vi "Write LIV Test data.vi"(7 "Send any changes now? (F)":bool, 8 "error in (no error)":errorcluster, 10 "LIV Test data":T1(array[cluster]), 11 "Fiber Auto Collimation state data in":refnum<class "Fiber Auto Collimation state data.lvclass">) -> (0 "error out":errorcluster, 3 "Fiber Auto Collimation state data out":refnum<class "Fiber Auto Collimation state data.lvclass">)   [LabVIEW 2018]
doc: "This \"LIV test data\" is just a placeholder and example for how real test data might be stored. This accessor plus its data in the state data class private control probably need to be removed or replaced with something to hold test data for the actual station."
uses:
  Fiber Auto Collimation state data.lvclass
  Tracked state data.ctl
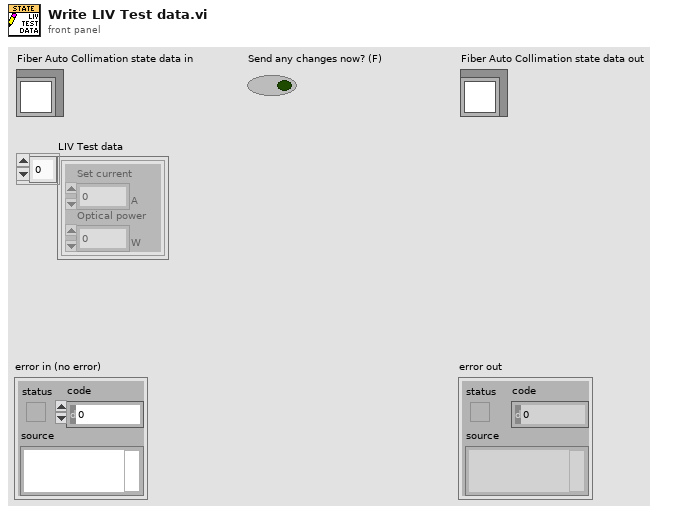
[diagram p1: front panel]
types:
  T1 = cluster{"Set current":sgl[unit], "Optical power":sgl[unit]}[]
  T2 = typedef "Fiber Auto Collimation state data.lvclass/Tracked state data.ctl" = enum16{"No update", "Permission level", "Username", "Test running", "DUT Serial", "Test status", "MOM Lot", "Loaded test recipe", "Model case running", "Station status", "BV data", "Defect Identify data", "Axis Position data", "Fiber Ass PN", "Operator", "RunTime", "VBAI", "Steps Cycle Time"}
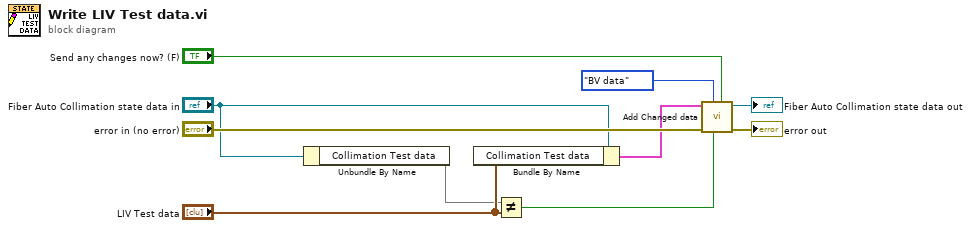
[diagram p0: block diagram]
diagram:
  n1 = Unbundle By Name("Fiber Auto Collimation state data in") -> ("Collimation Test data"=w2)
  n2 = Bundle By Name(cluster="Fiber Auto Collimation state data in", "Collimation Test data"="LIV Test data") -> (w6:cluster{})
  n3 = Not Equal?(x=w2, y="LIV Test data") -> (x != y?=w3:bool)
  n4 = call "Add Changed data.vi"("Send any changes now? (F)"="Send any changes now? (F)", "Data changed?"=w3, "Data type"=Tracked_state_data."BV data", "error in (no error)"="error in (no error)", "Fiber Auto Collimation state data in"=w6) -> ("error out"=→"error out":errorcluster, "Fiber Auto Collimation state data out"=→"Fiber Auto Collimation state data out":refnum<class "Fiber Auto Collimation state data.lvclass">)  [unwired: 5 in]
